vi "Abyss-watcher_luncher.vi"() -> ()   [LabVIEW 2021]
panel:
  out "Boolean 3":bool
  in  "Boolean 2":bool
  in  "Boolean":bool
  out "data out":dbl
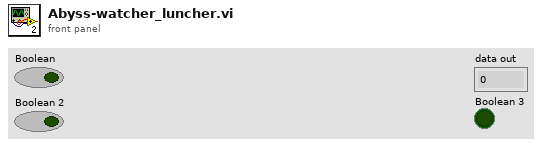
[diagram p1: front panel]
types:
  T1 = enum32{"Invalid", "Standard", "Closed", "Hidden", "Minimized", "Maximized"}
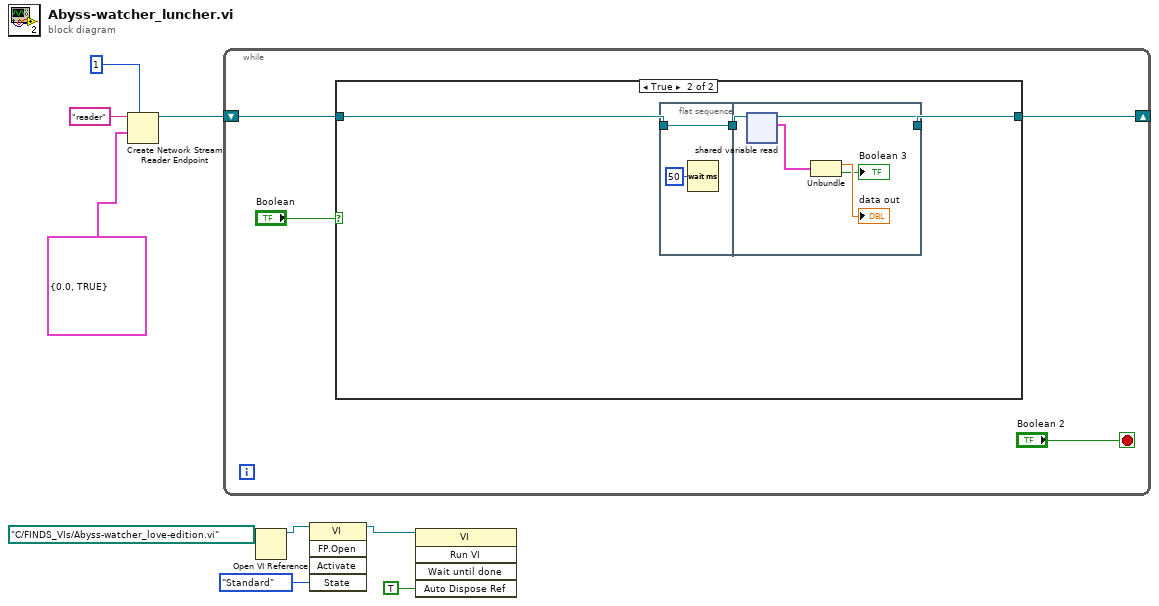
[diagram p0: block diagram]
diagram:
  n1 = Create Network Stream Reader Endpoint(7:1 ("reader buffer size"), 9:cluster{dbl, bool} {0.0, TRUE}, 11:"reader" ("reader name")) -> (3:w7:refnum<k21>)  [unwired: 4 in, 1 out]
  n2 = while {
    shift-right: [w12] -> _
    shift-left: w7 -> [w13]
    stop <- "Boolean 2" stop-if-true
    n3 = case shown="True" "Boolean" {
      tunnel: w13 -> [w14 w17]
      tunnel: [w14 w16] -> w12
      frame False {
      }
      frame True {
        n4 = flat-sequence {
          tunnel: w17 -> [w19]
          tunnel: [w19] -> w15
          tunnel: [w23] -> w16
          tunnel: w15 -> [w24]
          frame #0 {
            n5 = Wait (ms)(milliseconds to wait=u32 50) -> ()  [unwired: 1 out]
          }
          frame #1 {
            n6 = shared-variable-read(w24) -> (w23:refnum<k21>, w22:cluster{dbl, bool})  [unwired: 2 in, 2 out]
            n7 = Unbundle(w22) -> (→"data out":dbl, →"Boolean 3":bool)
          }
        }
      }
    }
  }
  n8 = Open VI Reference(vi path=path "C:/FINDS_VIs/Abyss-watcher_love-edition.vi") -> (vi reference=w5:refnum<vi>)  [unwired: 5 in, 1 out]
  n9 = invoke class="VI" method="FP.Open"(reference=w5, "State"=T1."Standard") -> (reference out=w3:refnum<vi>)  [unwired: 3 in, 4 out]
  n10 = invoke class="VI" method="Run VI"(reference=w3, "Auto Dispose Ref"=TRUE ("Auto Dispose Reference")) -> ()  [unwired: 3 in, 5 out]
